vi "Invoke Slot VI (Bool).vi"(4 "User Parameter":T1, 5 "Event Data":cluster{"Bool Value":bool}, 6 "User Event Ref":refnum<user-event>, 7 "Event Common Data":T3 {"Event Source" items=["LabVIEW UI"=0, "ActiveX"=1, "User Event"=25]}) -> ()   [LabVIEW 2013, in "Template.lvlib" / "LQCoreEngine.lvclass"]
uses:
  LQCoreEngine.lvclass
  <vilib>/event_ctls.llb/eventsource.ctl
  LQObject/LQObject.lvclass
panel:
  # "Copyright (c) 2016 Sze Howe Koh\n\nThis Source Code Form is subject to the terms of the Mozilla Public\nLicense, v. 2.0. If a copy of the MPL was not distributed with this\nfile, You can obtain one at http://mozilla.org/MPL/2.0/."
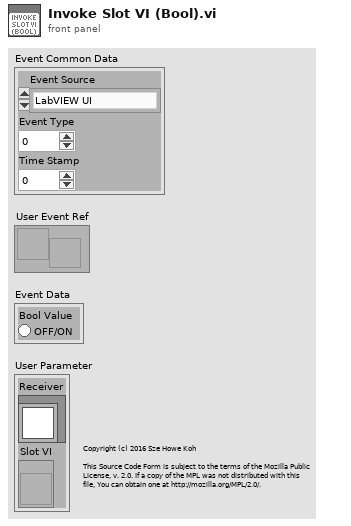
[diagram p1: front panel]
types:
  T1 = cluster{"Receiver":refnum<class "LQObject.lvclass">, "Slot VI":refnum<vi>}
  T2 = typedef "eventsource.ctl" = u32
  T3 = cluster{"Event Source":T2, "Event Type":u32, "Time Stamp":u32}
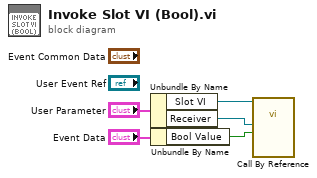
[diagram p0: block diagram]
diagram:
  n1 = Unbundle By Name("User Parameter") -> ("Slot VI"=w4:refnum<vi>, "Receiver"=w1:refnum<class "LQObject.lvclass">)
  n2 = Unbundle By Name("Event Data") -> ("Bool Value"=w2:bool)
  n3 = call-by-ref "?"(reference=w4, "Signal Parameter"=w2, "Receiver"=w1) -> ()  [unwired: 11 in, 2 out]
